vi "multiple_loops_safe.vi"() -> ()   [LabVIEW 2019]
panel:
  out "result":i32
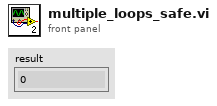
[diagram p1: front panel]
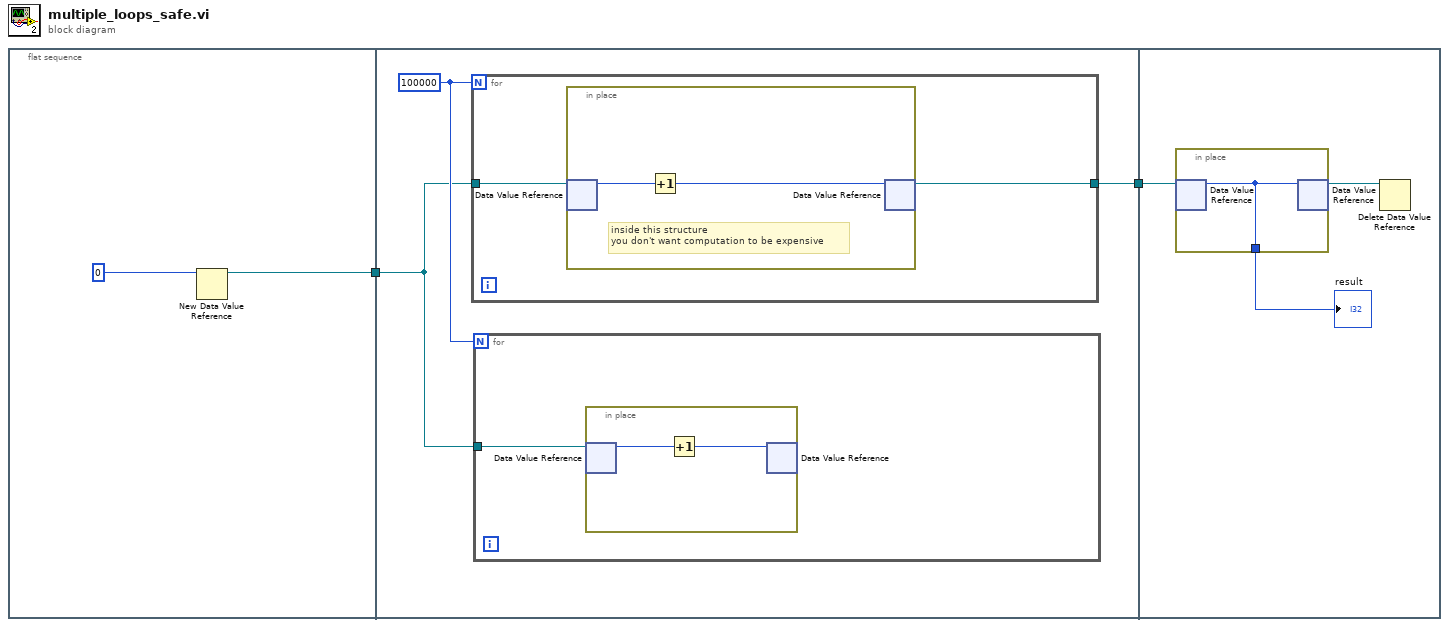
[diagram p0: block diagram]
diagram:
  n1 = flat-sequence {
    tunnel: [w3] -> w2
    tunnel: w2 -> [w6]
    tunnel: [w5] -> w1
    tunnel: w1 -> [w17]
    frame #0 {
      n2 = New Data Value Reference(data value=0) -> (data value reference=w3:refnum<data-value>)  [unwired: 1 in, 1 out]
    }
    frame #1 {
      w7 = 100000
      n3 = for {
        N: w7 -> [_]
        tunnel: w6 -> [w11]
        tunnel: [w12] -> w5
        n4 = in-place {
          # "inside this structure \nyou don't want computation to be expensive"
          n5 = in-place-dvr #1(w11) -> (w14:i32)  [unwired: 1 out]
          n6 = Increment(x=w14) -> (x+1=w13:i32)
          n7 = in-place-dvr #1(w13) -> (w12:refnum<data-value>)  [unwired: 1 out]
        }
      }
      n8 = for {
        N: w7 -> [_]
        tunnel: w6 -> [w8]
        n9 = in-place {
          n10 = in-place-dvr #2(w8) -> (w10:i32)  [unwired: 1 out]
          n11 = Increment(x=w10) -> (x+1=w9:i32)
          n12 = in-place-dvr #2(w9) -> ()  [unwired: 2 out]
        }
      }
    }
    frame #2 {
      n13 = in-place {
        in-place-border: [w18] -> w15
        n14 = in-place-dvr #3(w17) -> (w18:i32)  [unwired: 1 out]
        n15 = in-place-dvr #3(w18) -> (w16:refnum<data-value>)  [unwired: 1 out]
      }
      "result" <- w15
      n16 = Delete Data Value Reference(data value reference=w16) -> ()  [unwired: 1 in, 2 out]
    }
  }
